vi "VisObtainRequestEvents.vi"(7 "Set (T)/Get (F)":bool, 8 "Error":errorcluster[](array[cluster])) -> (0 "Error":errorcluster[](array[cluster]), 3 "VisRequestEvents":T1)   [LabVIEW 2018, in "Visualization.lvlib" / "VisualizeBase.lvclass"]
uses:
  VisualizeBase.lvclass
  VisRequestEvents.ctl
  VisUserEventType.ctl
  <userlib>/NIST/NISTErrorLib/NISTErrorLib.lvlib
panel:
  # "If you want to add other Request Events, open this typedef, copy an existing event and rename it to your event name."
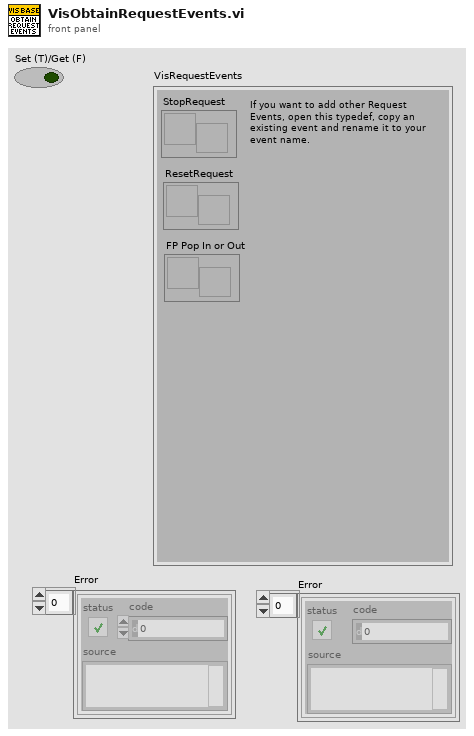
[diagram p1: front panel]
types:
  T1 = typedef "Visualization.lvlib/VisualizeBase.lvclass/VisRequestEvents.ctl" = cluster{"StopRequest":refnum<user-event>, "ResetRequest":refnum<user-event>, "FP Pop In or Out":refnum<user-event>}
  T2 = typedef "Visualization.lvlib/VisualizeBase.lvclass/VisUserEventType.ctl" = cluster{"BusIndex":i8, "Data":variant}
  T3 = typedef "Visualization.lvlib/VisualizeBase.lvclass/clRequestEvents.ctl" = cluster{"StopRequest":refnum<user-event>, "ResetRequest":refnum<user-event>, "FP Pop In or Out":refnum<user-event>}
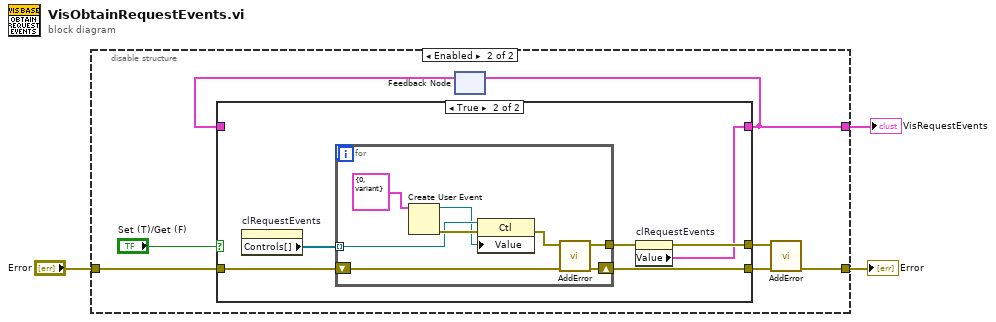
[diagram p0: block diagram]
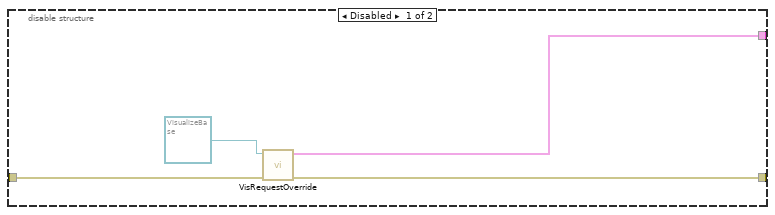
[diagram p2: hidden frame]
diagram:
  n1 = disable-structure shown="Enabled" {
    disable-tunnel: [w7 w8] -> w1
    disable-tunnel: "Error" -> [w6 w14]
    disable-tunnel: [w5 w11] -> w2
    frame Disabled {
      n2 = call-dynamic "VisRequestOverride.vi"("Error in"=w6, "Visualize"=refnum<class "VisualizeBase.lvclass"> refnum ("Visualization.lvlib:VisualizeBase_class.lvclass")) -> ("Error out"=w5:errorcluster[], "RequestEvents"=w7:T1)  [unwired: 8 in]
    }
    frame Enabled {
      n3 = feedback #1() -> (w9:T3)  [unwired: 1 in]
      n4 = case shown="True" "Set (T)/Get (F)" {
        tunnel: w14 -> [w15 w22]
        tunnel: [_ w18] -> w13
        tunnel: [w15 w21] -> w12
        tunnel: [w16 w17] -> w8
        tunnel: w9 -> [w16 _]
        frame False {
        }
        frame True {
          n5 = property on="clRequestEvents" class="Clust (strict)"() -> ("Controls[]"=w20:refnum<vi>[])  [unwired: 2 in, 2 out]
          n6 = for {
            shift-right: [w27] -> w21
            shift-left: w22 -> [w28]
            tunnel: [w26] -> w19
            tunnel: w20 -> [w24] mode=indexing
            n7 = Create User Event(user event datatype=T2 {"BusIndex"=0, "Data"=variant} ("clEventType")) -> (user event=w23:refnum<user-event>, error out=w29:errorcluster)  [unwired: 1 in]
            n8 = property class="Ctl"(reference=w24, error in=w29, "Value"=w23) -> (error out=w25:errorcluster)  [unwired: 1 out]
            n9 = call <userlib>:"AddError.vi"("ErrorArray In"=w28, "error in (no error)"=w25) -> ("ErrorArray Out"=w27:errorcluster[], "error out"=w26:errorcluster)  [unwired: 8 in]
          }
          n10 = property on="clRequestEvents" class="Clust (strict)"(error in=w19) -> (error out=w18:errorcluster, "Value"=w17:T3)  [unwired: 1 in, 1 out]
        }
      }
      n11 = feedback-in #1(w8) -> ()
      n12 = call <userlib>:"AddError.vi"("ErrorArray In"=w12, "error in (no error)"=w13) -> ("ErrorArray Out"=w11:errorcluster[])  [unwired: 8 in, 1 out]
    }
  }
  "VisRequestEvents" <- w1
  "Error" <- w2
